vi "Array_doppelte_Werte_entfernen.vi"(11 "Array":dbl[](array[numeric])) -> (2 "Indizes des doppelten Elemente":i32[](array[numeric])=[1, 4, 6, 7, 10], 3 "Array ohne Duplikate":dbl[](array[numeric]))   [LabVIEW 2012]
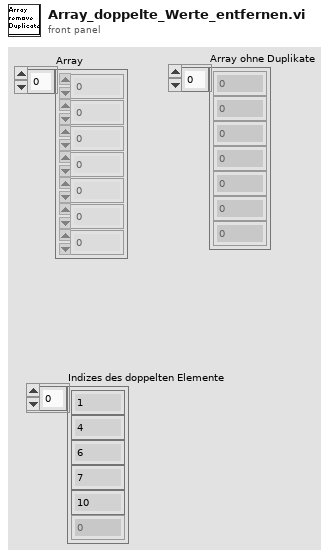
[diagram p1: front panel]
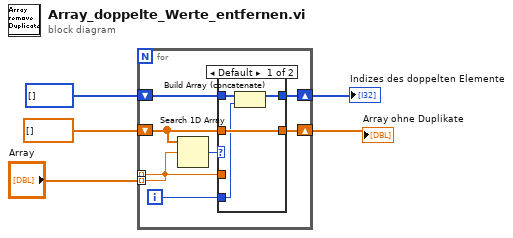
[diagram p0: block diagram]
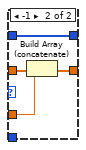
[diagram p2: hidden frame]
diagram:
  n1 = for {
    tunnel: [w6] -> _ mode=indexing
    shift-right: [w11] -> w1
    shift-left: dbl[] [] -> [w10]
    shift-right: [w8] -> w5
    shift-left: i32[] [] -> [w7]
    tunnel: "Array" -> [w6] mode=indexing
    i -> [w9]
    n2 = Search 1D Array(1D array=w10, element=w6) -> (index of element=w12:i32)  [unwired: 1 out]
    n3 = case shown="Default" w12 {
      tunnel: w6 -> [_ w20]
      tunnel: [w16 w18] -> w11
      tunnel: w10 -> [w16 w19]
      tunnel: w9 -> [w13 _]
      tunnel: [w14 w17] -> w8
      tunnel: w7 -> [w15 w17]
      frame Default {
        n4 = Build Array (concatenate)(w15, w13) -> (w14:i32[])
      }
      frame -1 {
        n5 = Build Array (concatenate)(w19, w20) -> (w18:dbl[])
      }
    }
  }
  "Indizes des doppelten Elemente" <- w5
  "Array ohne Duplikate" <- w1
